vi "Day 7 - Camel Cards.vi"() -> ()   [LabVIEW 2020, in "AoC 2023.lvlib"]
uses:
  AoC 2023.lvlib
panel:
  out "Puzzle Part-2 Answer":string
  out "Puzzle Answer":string
  in  "Puzzle Input":string="32T3K 765\nT55J5 684\nKK677 28\nKTJJT 220\nQQQJA 483"
  # "Enter the Puzzle Input and run the VI"
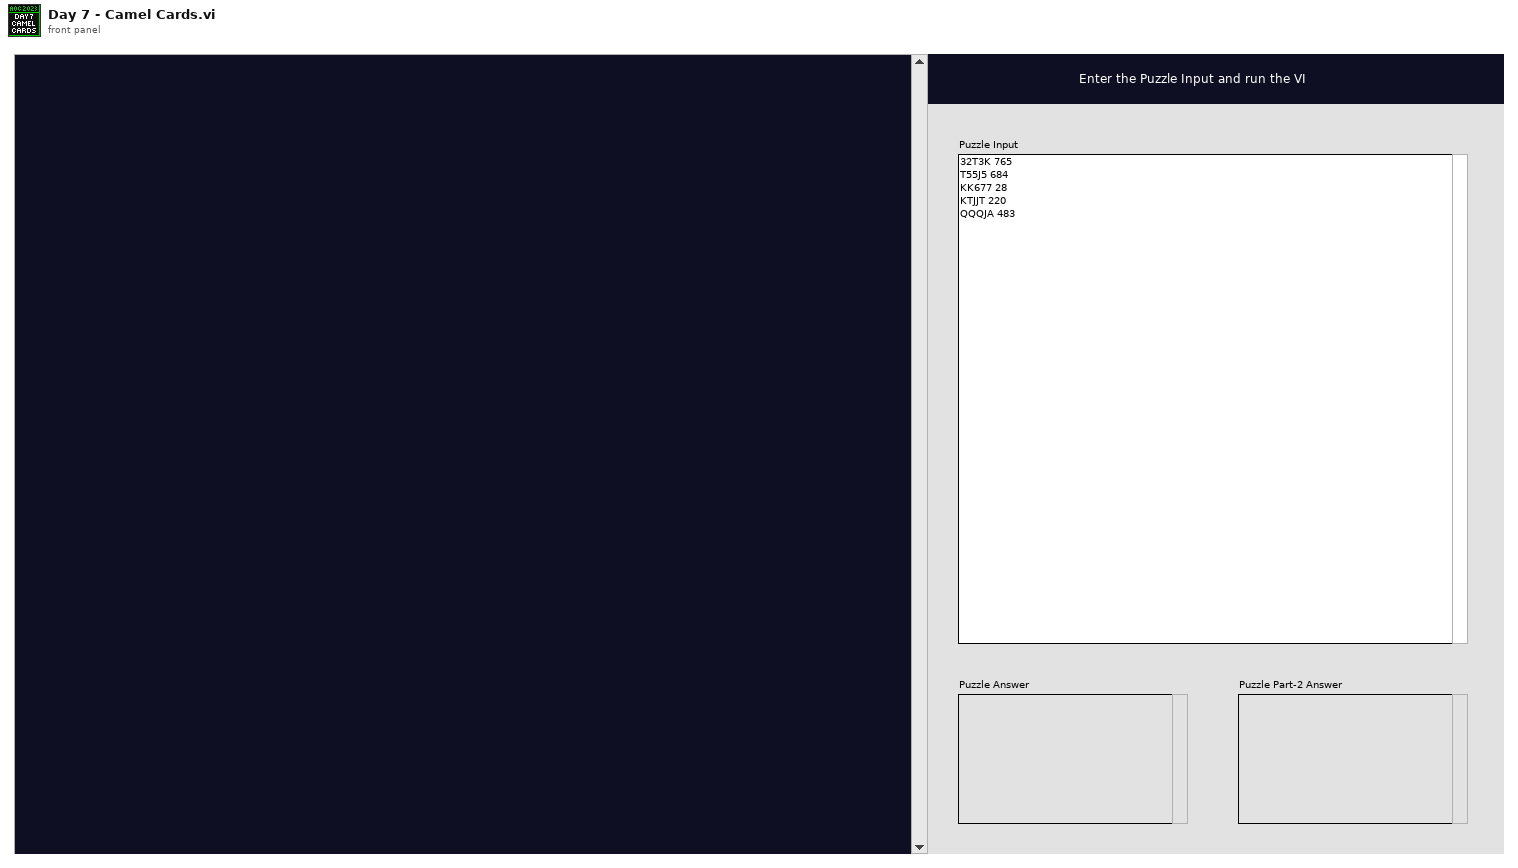
[diagram p1: front panel]
types:
  T1 = typedef "AoC 2023.lvlib/Type of a Hand.ctl" = enum16{"High card", "One pair", "Two pair", "Three of a kind", "Full house", "Four of a kind", "Five of a kind", "Unknown"}
  T2 = cluster{"Type":T1, "Strength of a Hand":i32[], i32, string, i32}
  T3 = cluster{"Type":T1, "Strength of a Hand":i32[], i32, string, i32}[]
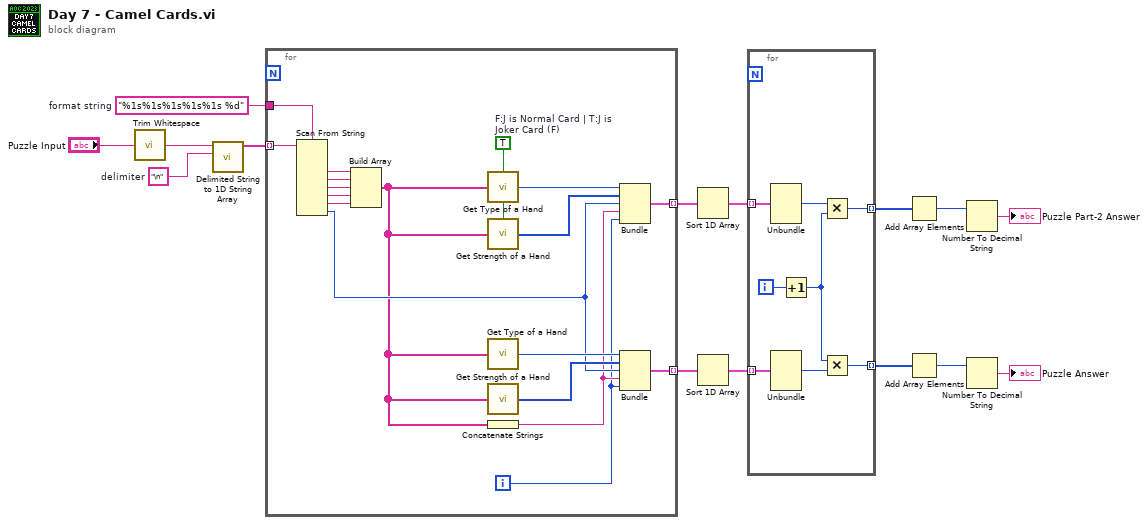
[diagram p0: block diagram]
diagram:
  w10 = "%1s%1s%1s%1s%1s %d"  # format string
  w12 = "\n"  # delimiter
  n1 = call <vilib>:"Trim Whitespace.vi"("string"="Puzzle Input") -> ("trimmed string"=w9:string)  [unwired: 1 in]
  n2 = call <vilib>:"Delimited String to 1D String Array.vi"("delimiter"=w12, "delimited string"=w9) -> ("string array"=w11:string[])  [unwired: 9 in]
  n3 = for {
    tunnel: w11 -> [w33] mode=indexing
    tunnel: w10 -> [w32]
    tunnel: [w26] -> w8 mode=indexing
    tunnel: [w21] -> w4 mode=indexing
    i -> [w16]
    w17 = TRUE  # F:J is Normal Card | T:J is Joker Card (F)
    n4 = Scan From String(format string=w32, input string=w33) -> (output 1=w31:string, output 2=w30:string, output 3=w29:string, output 4=w28:string, output 5=w27:string, output 6=w22:i32)  [unwired: 8 in, 3 out]
    n5 = Build Array(w31, w30, w29, w28, w27) -> (w19:string[])
    n6 = call "Get Type of a Hand.vi"("Cards in a hand"=w19, "F:J is Normal Card | T:J is Joker Card (F)"=w17) -> ("Type"=w24:T1)
    n7 = call "Get Strength of a Hand.vi"("Cards in a hand"=w19, "F:J is Normal Card | T:J is Joker Card (F)"=w17) -> ("Strength of a Hand"=w20:i32[])
    n8 = call "Get Type of a Hand.vi"("Cards in a hand"=w19) -> ("Type"=w25:T1)  [unwired: 1 in]
    n9 = call "Get Strength of a Hand.vi"("Cards in a hand"=w19) -> ("Strength of a Hand"=w23:i32[])  [unwired: 1 in]
    n10 = Concatenate Strings(w19) -> (w18:string)
    n11 = Bundle("Type"=w24, "Strength of a Hand"=w20, w22, w18, w16) -> (w21:T2)  [unwired: 1 in]
    n12 = Bundle("Type"=w25, "Strength of a Hand"=w23, w22, w18, w16) -> (w26:T2)  [unwired: 1 in]
  }
  n13 = Sort 1D Array(array=w4) -> (sorted array=w3:T3)
  n14 = Sort 1D Array(array=w8) -> (sorted array=w5:T3)
  n15 = for {
    tunnel: w5 -> [w41] mode=indexing
    tunnel: [w39] -> w7 mode=indexing
    tunnel: w3 -> [w36] mode=indexing
    tunnel: [w34] -> w2 mode=indexing
    i -> [w40]
    n16 = Unbundle(w36) -> (w37:i32)  [unwired: 4 out]
    n17 = Unbundle(w41) -> (w38:i32)  [unwired: 4 out]
    n18 = Increment(x=w40) -> (x+1=w35:i32)
    n19 = Multiply(x=w37, y=w35) -> (x*y=w34:i32)
    n20 = Multiply(x=w35, y=w38) -> (x*y=w39:i32)
  }
  n21 = Add Array Elements(numeric array=w2) -> (sum=w1:i32)
  n22 = Add Array Elements(numeric array=w7) -> (sum=w6:i32)
  n23 = Number To Decimal String(number=w1) -> (decimal integer string=→"Puzzle Part-2 Answer":string)  [unwired: 1 in]
  n24 = Number To Decimal String(number=w6) -> (decimal integer string=→"Puzzle Answer":string)  [unwired: 1 in]
